vi "GRAPH DATA.vi"(7 "frequency":dbl=10.0 format="%0.2p", 8 "error in (no error)":errorcluster, 9 "amplitude":dbl=1.0 format="%0.2p", 10 "signal type":T1(ring), 11 "SEÑAL_ACTUALIZABLE in":refnum<class "  SEÑAL_ACTUALIZABLE.lvclass">) -> (0 "error out":errorcluster, 3 "SEÑAL_ACTUALIZABLE out":refnum<class "  SEÑAL_ACTUALIZABLE.lvclass">)   [LabVIEW 2019, in "  SEÑAL_ACTUALIZABLE.lvlib" / "  SEÑAL_ACTUALIZABLE.lvclass"]
uses:
  <vilib>/measure/NI_MABase.lvlib
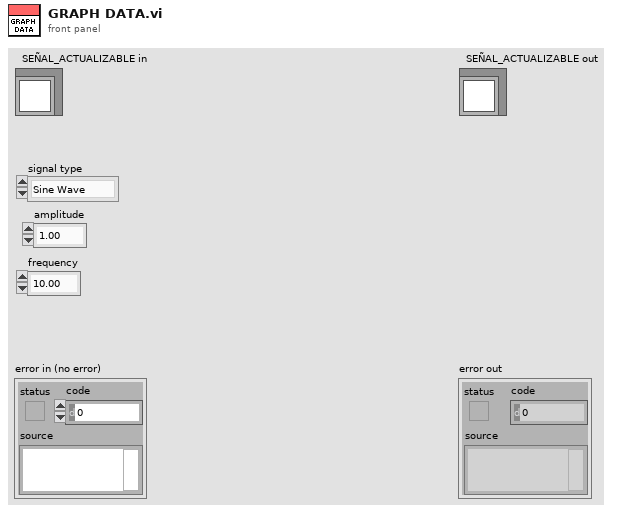
[diagram p1: front panel]
types:
  T1 = enum16{"Sine Wave", "Triangle Wave", "Square Wave", "Sawtooth Wave"}
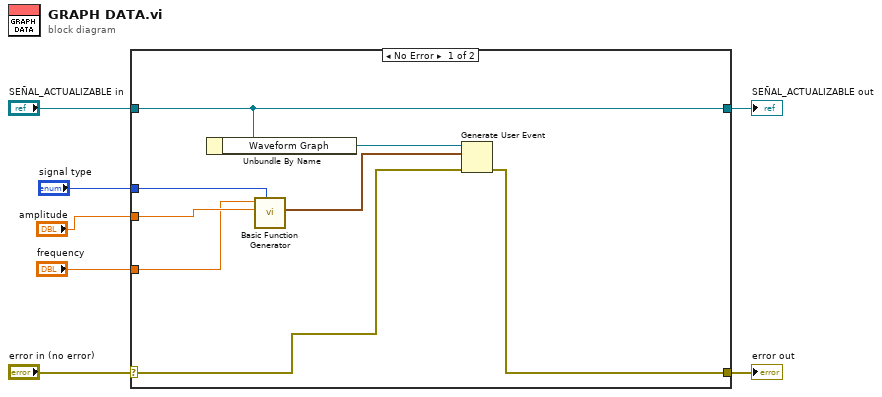
[diagram p0: block diagram]
diagram:
  n1 = case shown="No Error" "error in (no error)" {
    selector: "error in (no error)" -> [w9 w17]
    tunnel: [w8 w17] -> w6
    tunnel: [w15 w16] -> w4
    tunnel: "SEÑAL_ACTUALIZABLE in" -> [w15 w16]
    tunnel: "signal type" -> [w13 _]
    tunnel: "amplitude" -> [w12 _]
    tunnel: "frequency" -> [w11 _]
    frame No Error {
      n2 = Unbundle By Name(w15) -> ("Waveform Graph"=w14:refnum<user-event>)
      n3 = call <vilib>:"Basic Function Generator.vi"("signal type"=w13, "amplitude"=w12, "frequency"=w11) -> ("signal out"=w10:waveform(dbl))  [unwired: 6 in, 2 out]
      n4 = Generate User Event(user event=w14, event data cluster=w10, error in=w9) -> (error out=w8:errorcluster)  [unwired: 1 in, 1 out]
    }
    frame Error {
    }
  }
  "error out" <- w6
  "SEÑAL_ACTUALIZABLE out" <- w4
